vi "Corr Digitizer Reload.vi"(8 "error in (no error)":errorcluster, 11 "digitizer corrections in":T1) -> (0 "error out":errorcluster, 3 "digitizer corrections out":T1)   [LabVIEW 2013]
doc: "Takes correction path from the correction session and tries to load the digitizer corrections file. If the path is empty it will clear all the correction data in the correction session (blank correction)."
uses:
  Corr Digitizers.ctl
  octave/infolib.lvlibp/Private/Get key polymorph parts/GetString.vi
  octave/infolib.lvlibp/Private/Get matrix polymorph parts/Get 1D String.vi
  <vilib>/Utility/error.llb/Error Cluster From Error Code.vi
  <vilib>/ErrorRing/Error Ring.xnode
  octave/infolib.lvlibp
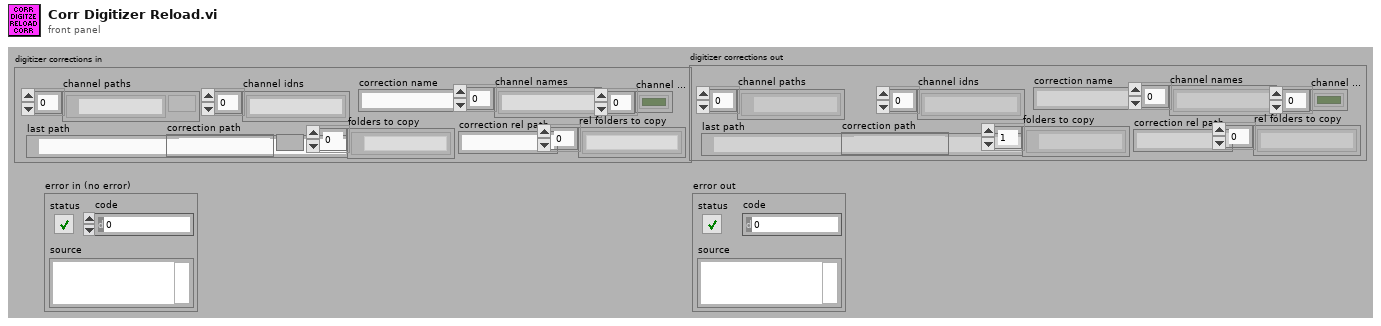
[diagram p1: front panel]
types:
  T1 = typedef "Corr Digitizers.ctl" = cluster{"last path":path, "channel paths":path[], "channel idns":string[], "correction name":string, "channel names":string[], "folders to copy":path[], "channel valid":bool[], "correction path":path, "correction rel path":string, "rel folders to copy":string[]}
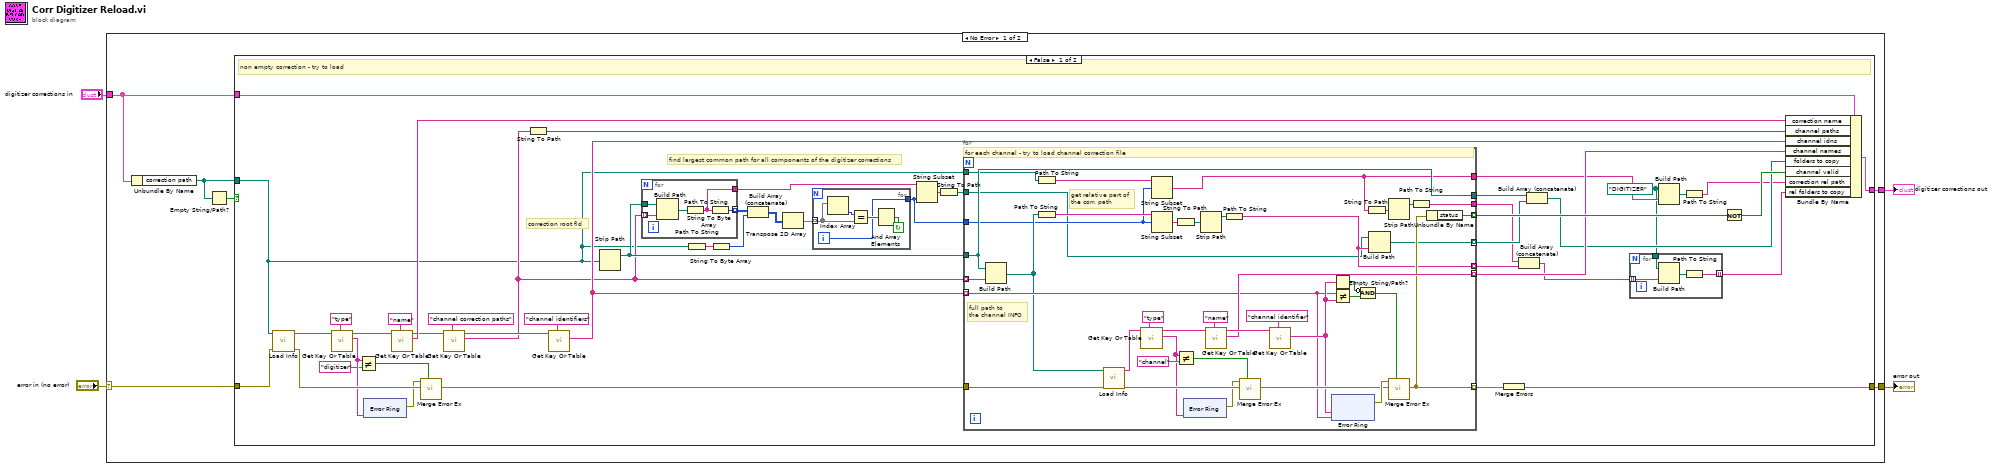
[diagram p0: block diagram]
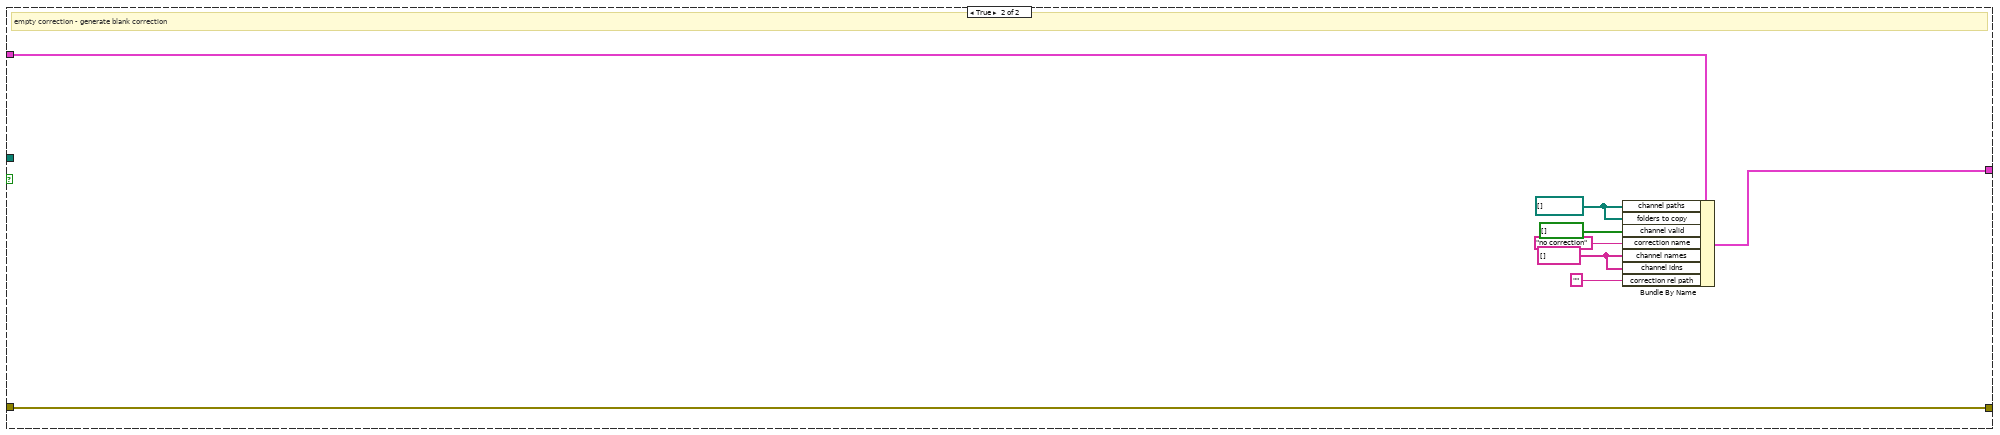
[diagram p2: hidden frame]
diagram:
  n1 = case shown="No Error" "error in (no error)" {
    selector: "error in (no error)" -> [w7 w142]
    tunnel: [w10 w142] -> w4
    tunnel: [w9 w143] -> w3
    tunnel: "digitizer corrections in" -> [w8 w143]
    frame No Error {
      n2 = Unbundle By Name(w8) -> ("correction path"=w5:path)
      n3 = Empty String/Path?(string/path=w5) -> (empty?=w6:bool)
      n4 = case shown="False" w6 {
        tunnel: [w58 w141] -> w10
        tunnel: [w57 w136] -> w9
        tunnel: w8 -> [w35 w140]
        tunnel: w5 -> [w21 _]
        tunnel: w7 -> [w34 w141]
        frame False {
          w12 = path "DIGITIZER" ("base path")
          # "find largest common path for all components of the digitizer corrections"
          # "correction root fld"
          # "non empty correction - try to load"
          n5 = call "Load Info.vi"("error in"=w34, "filename"=w21) -> ("error out"=w49:errorcluster, "info data"=w36:string)  [unwired: 8 in]
          n6 = call-poly "Get Key Or Table.vi"("key description"="type", "info data"=w36) -> ("value"=w40:string, "info data out"=w42:string)  [unwired: 6 in, 2 out]
          n7 = Not Equal?(x=w40, y="digitizer") -> (x != y?=w41:bool)
          n8 = xnode "Error Ring"("parameter 0"=w40) -> ("error out"=w39:errorcluster)
          n9 = call-poly "Get Key Or Table.vi"("key description"="name", "info data"=w42) -> ("value"=w47:string, "info data out"=w44:string)  [unwired: 6 in, 2 out]
          n10 = call "Merge Error Ex.vi"("Is error? (False)"=w41, "main error in (no error)"=w49, "second error in"=w39) -> ("error out"=w50:errorcluster)  [unwired: 8 in]
          n11 = call-poly "Get Key Or Table.vi"("key description"="channel correction paths", "info data"=w44) -> ("value"=w28:string[], "info data out"=w48:string)  [unwired: 6 in, 2 out]
          n12 = String To Path(string=w28) -> (path=w51:path[])
          n13 = call-poly "Get Key Or Table.vi"("key description"="channel identifiers", "info data"=w48) -> ("value"=w52:string[])  [unwired: 6 in, 3 out]
          n14 = Strip Path(path=w21) -> (stripped path=w29:path)  [unwired: 1 out]
          n15 = for {
            tunnel: w29 -> [w72]
            tunnel: w28 -> [w71] mode=indexing
            tunnel: [w68] -> w26
            tunnel: [w69] -> w25 mode=indexing
            n16 = Build Path(base path=w72, name or relative path=w71) -> (appended path=w70:path)
            n17 = Path To String(path=w70) -> (string=w68:string)
            n18 = String To Byte Array(string=w68) -> (unsigned byte array=w69:u8[])
          }
          n19 = Path To String(path=w21) -> (string=w23:string)
          n20 = String To Byte Array(string=w23) -> (unsigned byte array=w22:u8[])
          n21 = Build Array (concatenate)(w25, w22) -> (w24:u8[][])
          n22 = Transpose 2D Array(2D array=w24) -> (transposed array=w27:u8[][])
          n23 = for {
            tunnel: w27 -> [w66] mode=indexing
            tunnel: [w63] -> w18
            i -> [w63]
            stop <- w64 continue-if-true
            n24 = Index Array(array=w66) -> (element=w67:u8)  [unwired: 1 in]
            n25 = Equal?(x=w67, y=w66) -> (x = y?=w65:bool[])
            n26 = And Array Elements(Boolean array=w65) -> (logical AND=w64:bool)
          }
          n27 = String Subset(string=w26, length (rest)=w18) -> (substring=w20:string)  [unwired: 1 in]
          n28 = String To Path(string=w20) -> (path=w19:path)
          n29 = for {
            tunnel: w50 -> [w111]
            tunnel: w29 -> [w87]
            tunnel: w28 -> [w110] mode=indexing
            tunnel: w52 -> [w91] mode=indexing
            tunnel: [w96] -> w54 mode=indexing
            tunnel: [w90] -> w53 mode=indexing
            tunnel: [w89] -> w55 mode=indexing
            tunnel: [w88] -> w32 mode=indexing
            tunnel: [w87] -> w33
            tunnel: [w86] -> w15
            tunnel: w21 -> [w74]
            tunnel: [w83] -> w31
            tunnel: [w79] -> w30 mode=indexing
            tunnel: w19 -> [w73]
            tunnel: w18 -> [w76]
            # "get relative part of\nthe corr. path"
            # "full path to\nthe channel INFO"
            # "for each channel - try to load channel correction file"
            n30 = Build Path(base path=w87, name or relative path=w110) -> (appended path=w78:path)
            n31 = Path To String(path=w74) -> (string=w75:string)
            n32 = Path To String(path=w78) -> (string=w77:string)
            n33 = call "Load Info.vi"("error in"=w111, "filename"=w78) -> ("error out"=w106:errorcluster, "info data"=w109:string)  [unwired: 8 in]
            n34 = call-poly "Get Key Or Table.vi"("key description"="type", "info data"=w109) -> ("value"=w103:string, "info data out"=w102:string)  [unwired: 6 in, 2 out]
            n35 = String Subset(string=w75, offset (0)=w76) -> (substring=w86:string)  [unwired: 1 in]
            n36 = String Subset(string=w77, offset (0)=w76) -> (substring=w82:string)  [unwired: 1 in]
            n37 = String To Path(string=w82) -> (path=w81:path)
            n38 = Not Equal?(x=w103, y="channel") -> (x != y?=w104:bool)
            n39 = xnode "Error Ring"("parameter 0"=w103) -> ("error out"=w105:errorcluster)
            n40 = Strip Path(path=w81) -> (stripped path=w80:path)  [unwired: 1 out]
            n41 = call-poly "Get Key Or Table.vi"("key description"="name", "info data"=w102) -> ("value"=w96:string, "info data out"=w99:string)  [unwired: 6 in, 2 out]
            n42 = Path To String(path=w80) -> (string=w79:string)
            n43 = call "Merge Error Ex.vi"("Is error? (False)"=w104, "main error in (no error)"=w106, "second error in"=w105) -> ("error out"=w94:errorcluster)  [unwired: 8 in]
            n44 = call-poly "Get Key Or Table.vi"("key description"="channel identifier", "info data"=w99) -> ("value"=w92:string)  [unwired: 6 in, 3 out]
            n45 = xnode "Error Ring"("parameter 0"=w92, "parameter 1"=w91) -> ("error out"=w95:errorcluster)
            n46 = Empty String/Path?(string/path=w92) -> (empty?=w97:bool)
            n47 = Not Equal?(x=w91, y=w92) -> (x != y?=w98:bool)
            n48 = Compound Arithmetic op=AND(invert w97, w98) -> (w93:bool)
            n49 = String To Path(string=w86) -> (path=w85:path)
            n50 = Build Path(base path=w73, name or relative path=w79) -> (appended path=w88:path)
            n51 = call "Merge Error Ex.vi"("Is error? (False)"=w93, "main error in (no error)"=w94, "second error in"=w95) -> ("error out"=w90:errorcluster)  [unwired: 8 in]
            n52 = Strip Path(path=w85) -> (stripped path=w84:path)  [unwired: 1 out]
            n53 = Path To String(path=w84) -> (string=w83:string)
            n54 = Unbundle By Name(w90) -> ("status"=w89:bool)
          }
          n55 = Merge Errors(w53) -> (w58:errorcluster)
          n56 = Build Array (concatenate)(w31, w30) -> (w13:string[])
          n57 = Build Array (concatenate)(w33, w32) -> (w17:path[])
          n58 = for {
            tunnel: w13 -> [w60] mode=indexing
            tunnel: w12 -> [w61]
            tunnel: [w59] -> w11 mode=indexing
            n59 = Build Path(base path=w61, name or relative path=w60) -> (appended path=w62:path)
            n60 = Path To String(path=w62) -> (string=w59:string)
          }
          n61 = Build Path(base path=w12, name or relative path=w15) -> (appended path=w16:path)
          n62 = Path To String(path=w16) -> (string=w14:string)
          n63 = Not(x=w55) -> (.not. x?=w56:bool[])
          n64 = Bundle By Name(cluster=w35, "correction name"=w47, "channel paths"=w51, "channel idns"=w52, "channel names"=w54, "folders to copy"=w17, "channel valid"=w56, "correction rel path"=w14, "rel folders to copy"=w11) -> (w57:T1)
        }
        frame True {
          w135 = string[] [] ("channel names")
          w139 = path[] [] ("channel paths")
          # "empty correction - generate blank correction"
          n65 = Bundle By Name(cluster=w140, "channel paths"=w139, "folders to copy"=w139, "channel valid"=bool[] [], "correction name"="no correction", "channel names"=w135, "channel idns"=w135, "correction rel path"="") -> (w136:T1)
        }
      }
    }
    frame Error {
    }
  }
  "error out" <- w4
  "digitizer corrections out" <- w3
